vi "stop.vi"(8 "error in (no error)":errorcluster, 11 "Camera in":refnum<class "Camera.lvclass">) -> (0 "error out":errorcluster, 3 "Camera out":refnum<class "Camera.lvclass">)   [LabVIEW 2019, in "Camera.lvclass"]
doc: "Stops the current recording. In 'ring buffer' and 'fifo' mode, this function must be called\nby the user. In 'sequence' and 'sequence non blocking' mode, this function is automatically\ncalled when the number_of_images is reached."
uses:
  Camera.lvclass
  pco.recorder/Recorder.lvlib
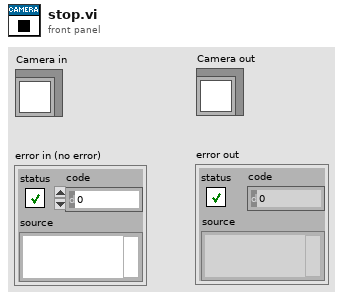
[diagram p1: front panel]
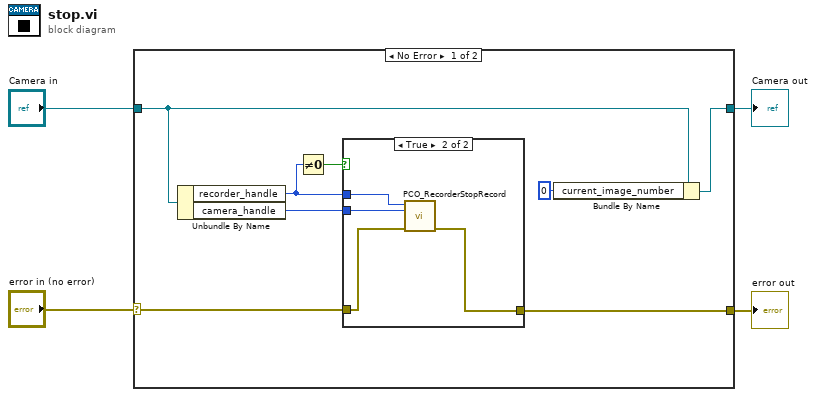
[diagram p0: block diagram]
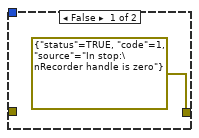
[diagram p2: hidden frame]
diagram:
  n1 = case shown="No Error" "error in (no error)" {
    selector: "error in (no error)" -> [w11 w19]
    tunnel: [w10 w19] -> w3
    tunnel: [w6 w18] -> w1
    tunnel: "Camera in" -> [w8 w18]
    frame No Error {
      n2 = Unbundle By Name(w8) -> ("recorder_handle"=w9:u64, "camera_handle"=w5:u64)
      n3 = Not Equal To 0?(x=w9) -> (x != 0?=w12:bool)
      n4 = case shown="True" w12 {
        tunnel: [errorcluster {"status"=TRUE, "code"=1, "source"="In stop:\nRecorder handle is zero"} ("error constant") w15] -> w10
        tunnel: w9 -> [_ w16]
        tunnel: w11 -> [_ w17]
        tunnel: w5 -> [_ w14]
        frame False {
        }
        frame True {
          n5 = call "PCO_RecorderStopRecord.vi"("error in (no error)"=w17, "phCam"=w14, "phRec"=w16) -> ("error out"=w15:errorcluster)  [unwired: 6 in, 2 out]
        }
      }
      n6 = Bundle By Name(cluster=w8, "current_image_number"=u32 0 ("current_image_index")) -> (w6:refnum<class "Camera.lvclass">)
    }
    frame Error {
    }
  }
  "error out" <- w3
  "Camera out" <- w1
